vi "Check Device Type.vi"(8 "error in (no error)":errorcluster, 9 "Device Type Name":string, 10 "DC Brick in":refnum<class "DC Brick.lvclass">) -> (0 "error out":errorcluster, 1 "correct Device":bool, 2 "DC Brick out":refnum<class "DC Brick.lvclass">)   [LabVIEW 2011, in "Tinkerforge.lvlib" / "DC Brick.lvclass"]
doc: "This VI is the child implementation of \"Check Device Type.vi\" and invokes the device type validation through checking the device name."
uses:
  DC Brick.lvclass
  Device/Device.lvclass
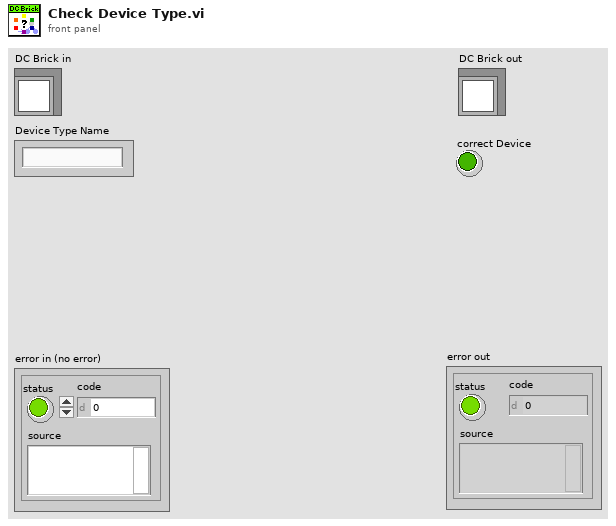
[diagram p1: front panel]
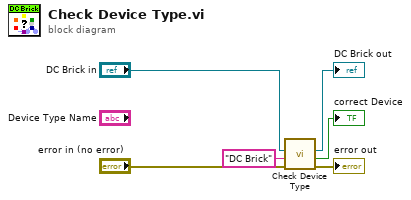
[diagram p0: block diagram]
diagram:
  n1 = call-parent "Check Device Type.vi"("error in (no error)"="error in (no error)", "Device Type Name"="DC Brick", "Device in"="DC Brick in") -> ("error out"=→"error out":errorcluster, "correct Device"=→"correct Device":bool, "Device out"=→"DC Brick out":refnum<class "DC Brick.lvclass">)  [unwired: 6 in]
